vi "Byte Buffer.Write (Pointer).vi"(7 "count":i64, 8 "error in (no error)":errorcluster, 9 "src pointer":u64, 10 "buffer offset":u64, 11 "Byte Buffer in":refnum<class "Byte Buffer.lvclass">) -> (0 "error out":errorcluster, 2 "new buffer offset":u64, 3 "Byte Buffer out":refnum<class "Byte Buffer.lvclass">)   [LabVIEW 2016, in "VeriStand Data.lvlib" / "Byte Buffer.lvclass"]
doc: "Writes data of size <B>bytes to copy</B> from the memory location specified by <B>src pointer</B> to the provided <B>Byte Buffer</B> at location <B>buffer offset</B>."
uses:
  Byte Buffer.lvclass
  Byte Buffer.lvclass/Byte Buffer.ctl
  Memory Management/Memory Management.Handle Return.vi
  VeriStand Data.lvlib
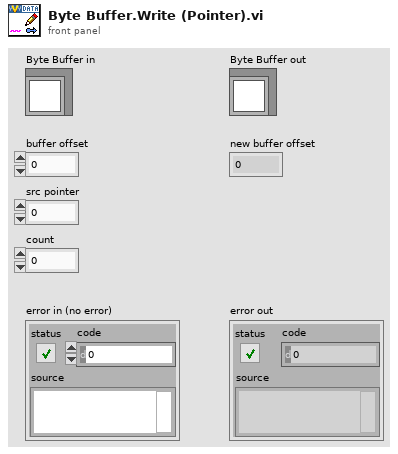
[diagram p1: front panel]
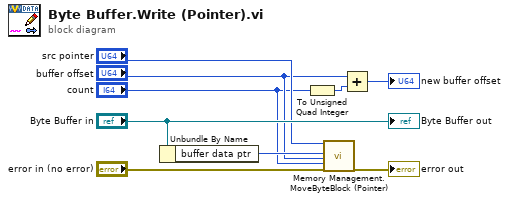
[diagram p0: block diagram]
diagram:
  n1 = Unbundle By Name("Byte Buffer in") -> ("buffer data ptr"=w5:u64)
  n2 = To Unsigned Quad Integer(1:"count") -> (0:w3:u64)
  n3 = call "Memory Management.MoveByteBlock (Pointer).vi"("src ptr in"="src pointer", "dst ptr in"=w5, "dst offset (0)"="buffer offset", "size"="count", "error in (no error)"="error in (no error)") -> ("error out"=→"error out":errorcluster)  [unwired: 9 in, 5 out]
  n4 = Add(x="buffer offset", y=w3) -> (x+y=→"new buffer offset":u64)
  "Byte Buffer out" <- "Byte Buffer in"
